vi "Page_Preview_Update_Tree_Icons.vi"(7 "Preview Tree":refnum<vi>, 8 "error in (no error)":errorcluster, 11 "AB_EXE in":refnum<class "AB_EXE.lvclass">) -> (0 "error out":errorcluster, 3 "AB_EXE out":refnum<class "AB_EXE.lvclass">)   [LabVIEW 2020, in "AB_EXE.lvclass"]
uses:
  <vilib>/AppBuilder/AB_Classes/EXE/AB_EXE.lvclass
  e:/builds/penguin/labview/branches/2020/dev/dist/vi.lib/AppBuilder/AB_Classes/Build/AB_Build.lvclass
  e:/builds/penguin/labview/branches/2020/dev/dist/vi.lib/AppBuilder/AB_Classes/TargetFile/AB_Targetfile.lvclass
  <vilib>/AppBuilder/AB_Classes/EXE/AB_EXE.lvclass/AB_EXE.ctl
  <vilib>/AppBuilder/AB_Classes/Destination/AB_Destination.lvclass
  <vilib>/AppBuilder/AB_Classes/Build/AB_Build.lvclass
  <vilib>/AppBuilder/AB_Classes/TargetFile/AB_Targetfile.lvclass
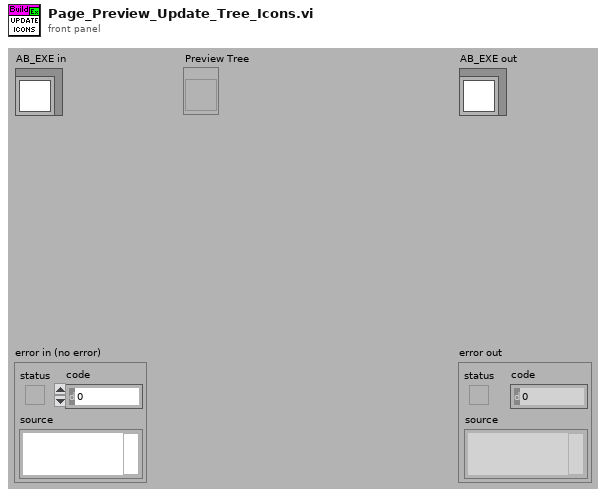
[diagram p1: front panel]
types:
  T1 = typedef "AB_Build.ctl" = cluster{"buildSpecName":string, "buildSpecDescription":string, "destinations":refnum<class "AB_Destination.lvclass">[], "exclusionOption":T2, "defaultLanguage":string, "supportedLanguages":string[], "excludedDirectories":path[], "buildContext":refnum<vi>, "buildObject":T3, "preview":bool, "programatic":bool, "progressBarEvents":T4, "userLog_Path":path, "preActionID":string, "preAction_Path":path, "postActionID":string, "postAction_Path":path, "eng_checkForBrokenVIs?":bool, "eng_verboseLinkerErrors?":bool, "localDest_Path":path, "targetDest_Path":path, "removeVIObject":u16, "cache":refnum<class "PreviewCache.lvclass">, "use cache":bool, "previewCache_ID":string, "buildCache_ID":string, "eng_TempLocalDest_Path":path, "eng_collectDependencies?":bool, "versionInfo":cluster{"buildVersion":cluster{"major":u16, "minor":u16, "patch":u16, "build":u16}, "autoIncrement":bool}, "eng_enableVIChecksums":bool}
  T2 = typedef "AB_Exclusion_Option.ctl" = cluster{"typedefs":bool, "polymorphicVIs":bool, "unusedLibraryItems":bool, "modifyLibraryFile":bool, "edit-timeDependencies":bool, "inlineVIs":bool, "dependent PPLs":bool, "dependent DLLs":bool}
  T3 = typedef "ItemRef.ctl" = u64
  T4 = typedef "provcom_ProgressBar_Events.ctl" = cluster{"newJob":refnum<user-event>, "newItem":refnum<user-event>, "errorMsg":T5, "cancel":refnum<user-event>}
  T5 = typedef "mxLvBuildError.ctl" = refnum<user-event>
  T6 = typedef "AB_Targetfile.ctl" = cluster{"targetfileName":string, "targetfileGUID":string, "enableDebugging":bool, "versionInfo":cluster{"productName":string, "legalCopyright":string, "companyName":string, "internalName":string, "fileDescription":string}, "eng_consolidatedTypeInfo":string, "fastFileFormat":bool, "eng_LEIFBuildData":u32, "versionIndependent":bool}
  T7 = typedef "AB_Destination.ctl" = cluster{"destName":string, "path":path, "libraryName":string, "preserveHierarchy":bool, "eng_inBuild":bool, "eng_libraryReference":refnum<vi>, "eng_restictAddToNewLibrary":bool}
  T8 = typedef "imagedata.ctl" = cluster{"image type":i32, "image depth":i32, "image":u8[], "mask":u8[], "colors":u32[], "Rectangle":cluster{"left":i16, "top":i16, "right":i16, "bottom":i16}}
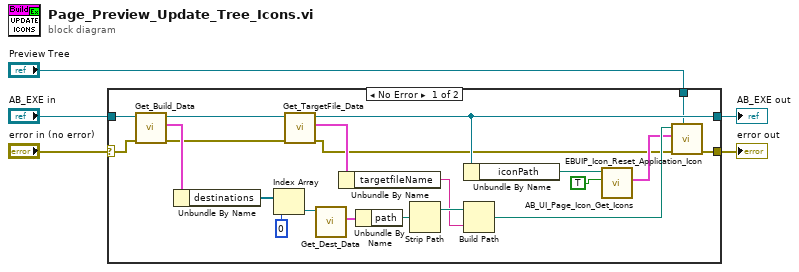
[diagram p0: block diagram]
diagram:
  n1 = case shown="No Error" "error in (no error)" {
    selector: "error in (no error)" -> [w9 w27]
    tunnel: "AB_EXE in" -> [w16 w28]
    tunnel: [w14 w28] -> w4
    tunnel: "Preview Tree" -> [w10 _]
    tunnel: [w6 w27] -> w1
    frame No Error {
      n2 = call <vilib>:"Get_Build_Data.vi"("error in (no error)"=w9, "Class in"=w16) -> ("error out"=w8:errorcluster, "data"=w26:T1, "Class out"=w15:refnum<class "AB_EXE.lvclass">)  [unwired: 7 out]
      n3 = Unbundle By Name(w26) -> ("destinations"=w25:refnum<class "AB_Destination.lvclass">[])
      n4 = Index Array(array=w25, index=0) -> (element=w21:refnum<class "AB_Destination.lvclass">)
      n5 = call <vilib>:"Get_TargetFile_Data.vi"("error in (no error)"=w8, "AB_Targetfile in"=w15) -> ("error out"=w7:errorcluster, "data"=w19:T6, "AB_Targetfile out"=w14:refnum<class "AB_EXE.lvclass">)  [unwired: 7 in]
      n6 = call <vilib>:"Get_Dest_Data.vi"("Class in"=w21) -> ("destName"=w22:T7)  [unwired: 1 in, 9 out]
      n7 = Unbundle By Name(w19) -> ("targetfileName"=w18:string)
      n8 = Unbundle By Name(w22) -> ("path"=w20:path)
      n9 = Strip Path(path=w20) -> (stripped path=w23:path)  [unwired: 1 out]
      n10 = Unbundle By Name(w14) -> ("iconPath"=w13:path)
      n11 = Build Path(base path=w23, name or relative path=w18) -> (appended path=w12:path)
      n12 = call <resource>:"AB_UI_Page_Icon_Get_Icons.vi"("preview?"=TRUE, "Icon path"=w13) -> ("preview image data"=w11:T8)  [unwired: 1 in, 8 out]
      n13 = call <resource>:"EBUIP_Icon_Reset_Application_Icon.vi"("Preview Tree"=w10, "error in (no error)"=w7, "Application Icon"=w11, "Application Path"=w12) -> ("error out"=w6:errorcluster)  [unwired: 7 out]
    }
    frame Error {
    }
  }
  "error out" <- w1
  "AB_EXE out" <- w4
